vi "ep_D to Y convert (Vector).vi"(8 "error in (no error)":errorcluster, 11 "one-cycle fundamental line voltage vectors":T2(array[cluster])) -> (0 "error out":errorcluster, 3 "one-cycle fundamental phase voltage vectors":T2(array[cluster]))   [LabVIEW 2014, in "NI_EP_Power Quality.lvlib"]
uses:
  <vilib>/addons/Electrical Power/PQ/NI_EP_Power Quality.lvlib
  <vilib>/addons/Electrical Power/PQ/Common/Controls/ep_AI Data Channel.ctl
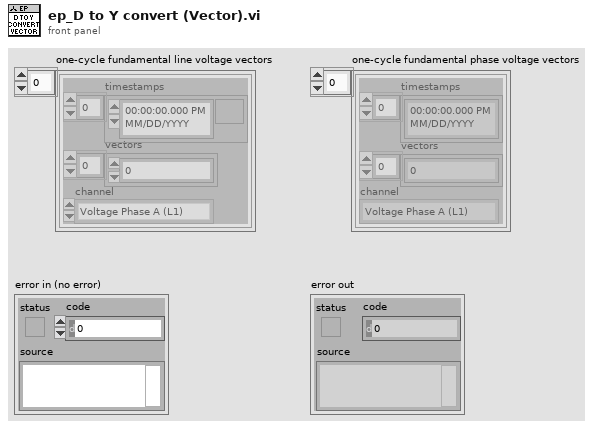
[diagram p1: front panel]
types:
  T1 = typedef "NI_EP_Power Quality.lvlib/ep_AI Data Channel.ctl" = enum16{"Voltage Phase A (L1)", "Voltage Phase B (L2)", "Voltage Phase C (L3)", "Voltage Phase N (Neutral)", "Current Phase A (L1)", "Current Phase B (L2)", "Current Phase C (L3)", "Current Phase N (Neutral)"}
  T2 = cluster{"timestamps":timestamp[], "vectors":cdb[], "channel":T1}[]
  T3 = cluster{"timestamps":timestamp[], "vectors":cdb[], "channel":T1}
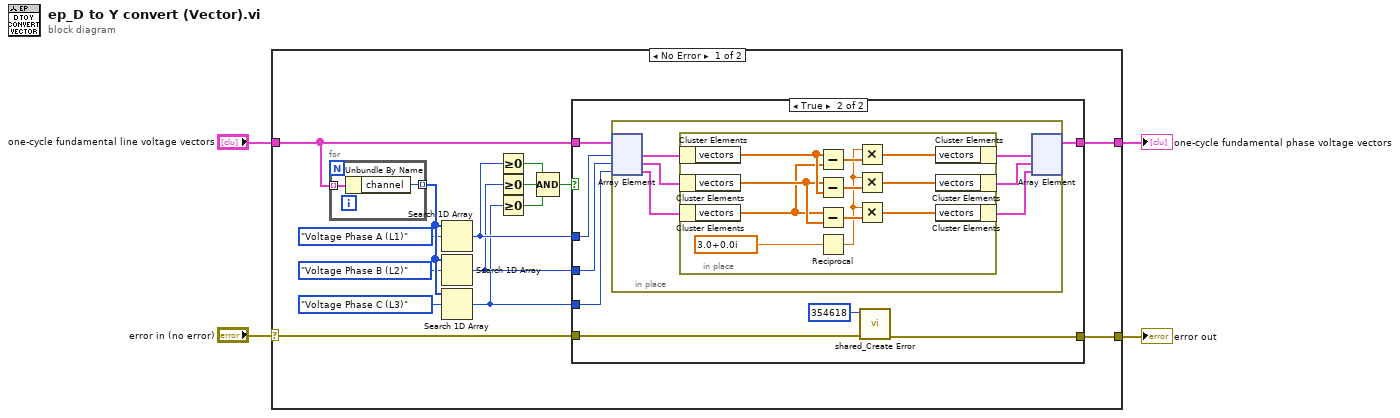
[diagram p0: block diagram]
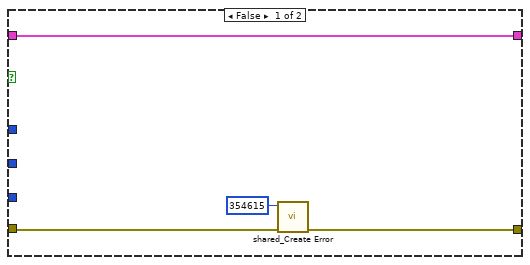
[diagram p2: hidden frame]
diagram:
  n1 = case shown="No Error" "error in (no error)" {
    selector: "error in (no error)" -> [w16 w52]
    tunnel: [w17 w52] -> w3
    tunnel: [w19 w51] -> w2
    tunnel: "one-cycle fundamental line voltage vectors" -> [w18 w51]
    frame No Error {
      n2 = for {
        tunnel: w18 -> [w21] mode=indexing
        tunnel: [w20] -> w13 mode=indexing
        n3 = Unbundle By Name(w21) -> ("channel"=w20:T1)
      }
      n4 = Search 1D Array(1D array=w13, element=ep_AI_Data_Channel."Voltage Phase A (L1)" ("AI data channel")) -> (index of element=w8:i32)  [unwired: 1 in]
      n5 = Search 1D Array(1D array=w13, element=ep_AI_Data_Channel."Voltage Phase B (L2)" ("AI data channel")) -> (index of element=w6:i32)  [unwired: 1 in]
      n6 = Search 1D Array(1D array=w13, element=ep_AI_Data_Channel."Voltage Phase C (L3)" ("AI data channel")) -> (index of element=w5:i32)  [unwired: 1 in]
      n7 = Greater Or Equal To 0?(x=w8) -> (x >= 0?=w9:bool)
      n8 = Greater Or Equal To 0?(x=w6) -> (x >= 0?=w14:bool)
      n9 = Greater Or Equal To 0?(x=w5) -> (x >= 0?=w15:bool)
      n10 = Compound Arithmetic op=AND(w9, w14, w15) -> (w7:bool)
      n11 = case shown="True" w7 {
        tunnel: [w25 w32] -> w19
        tunnel: w18 -> [w25 w33]
        tunnel: w8 -> [_ w31]
        tunnel: w6 -> [_ w30]
        tunnel: w5 -> [_ w29]
        tunnel: [w22 w28] -> w17
        tunnel: w16 -> [w23 w26]
        frame False {
          n12 = call <vilib>:"shared_Create Error.vi"("error in (no error)"=w23, "error code (0)"=354615) -> ("error out"=w22:errorcluster)  [unwired: 9 in]
        }
        frame True {
          n13 = in-place {
            n14 = in-place-array #1(w33, w31, w30, w29) -> (w39:T3, w38:T3, w37:T3)
            n15 = in-place {
              n16 = in-place-cluster #2(w39) -> ("vectors"=w45:cdb[])
              n17 = in-place-cluster #3(w38) -> ("vectors"=w44:cdb[])
              n18 = in-place-cluster #4(w37) -> ("vectors"=w43:cdb[])
              n19 = Subtract(x=w45, y=w43) -> (x-y=w49:cdb[])
              n20 = Subtract(x=w44, y=w45) -> (x-y=w48:cdb[])
              n21 = Subtract(x=w43, y=w44) -> (x-y=w47:cdb[])
              n22 = Reciprocal(x=cdb 3.0+0.0i) -> (1/x=w46:cdb)
              n23 = Multiply(x=w46, y=w49) -> (x*y=w40:cdb[])
              n24 = Multiply(x=w46, y=w48) -> (x*y=w41:cdb[])
              n25 = Multiply(x=w46, y=w47) -> (x*y=w42:cdb[])
              n26 = in-place-cluster #2("vectors"=w40) -> (w36:T3)
              n27 = in-place-cluster #3("vectors"=w41) -> (w35:T3)
              n28 = in-place-cluster #4("vectors"=w42) -> (w34:T3)
            }
            n29 = in-place-array #1(w36, w35, w34) -> (w32:T2)  [unwired: 3 out]
          }
          n30 = call <vilib>:"shared_Create Error.vi"("error in (no error)"=w26, "error code (0)"=354618) -> ("error out"=w28:errorcluster)  [unwired: 9 in]
        }
      }
    }
    frame Error {
    }
  }
  "one-cycle fundamental phase voltage vectors" <- w2
  "error out" <- w3
